vi "add_from_rio.vi"(4 "from_rio":T1, 5 "msg in":string) -> (2 "msg out":string)   [LabVIEW 2016]
uses:
  <userlib>/ROS for LabVIEW Software/ROS/MessageBuilding/std_msgs/subs/i8Scalar.vi
  <userlib>/ROS for LabVIEW Software/ROS/MessageBuilding/std_msgs/subs/stringScalar.vi
  <userlib>/ROS for LabVIEW Software/ROS/MessageBuilding/std_msgs/subs/timeScalar.vi
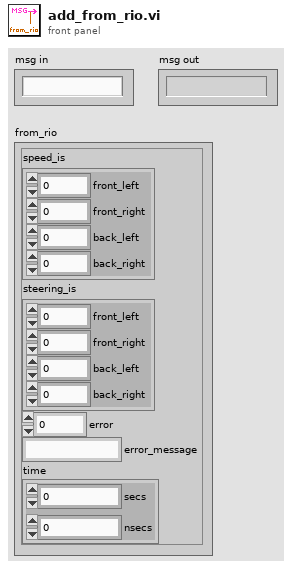
[diagram p1: front panel]
types:
  T1 = cluster{"speed_is":cluster{"front_left":dbl, "front_right":dbl, "back_left":dbl, "back_right":dbl}, "steering_is":cluster{"front_left":dbl, "front_right":dbl, "back_left":dbl, "back_right":dbl}, "error":i8, "error_message":string, "time":cluster{"secs":i32, "nsecs":i32}}
  T2 = cluster{"front_left":dbl, "front_right":dbl, "back_left":dbl, "back_right":dbl}
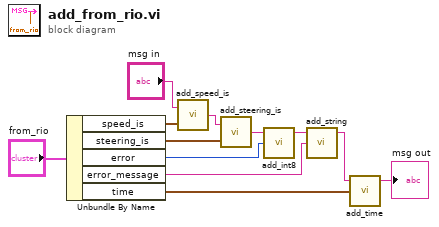
[diagram p0: block diagram]
diagram:
  n1 = Unbundle By Name("from_rio") -> ("speed_is"=w9:T2, "steering_is"=w8:T2, "error"=w7:i8, "error_message"=w6:string, "time"=w5:cluster{"secs":i32, "nsecs":i32})
  n2 = call "add_speed_is.vi"("speed_is"=w9, "msg in"="msg in") -> ("msg out"=w10:string)
  n3 = call "add_steering_is.vi"("steering_is"=w8, "msg in"=w10) -> ("msg out"=w4:string)
  n4 = call-poly <userlib>:"add_int8.vi"("Numeric"=w7, "msg in"=w4) -> ("msg out"=w3:string)  [unwired: 3 in]
  n5 = call-poly <userlib>:"add_string.vi"("String"=w6, "msg in"=w3) -> ("msg out"=w2:string)  [unwired: 3 in]
  n6 = call-poly <userlib>:"add_time.vi"("Time"=w5, "msg in"=w2) -> ("msg out"=→"msg out":string)  [unwired: 3 in]
